vi "External Actuator Calibrations DAO.vi"(7 "refnum":T2, 8 "error in (no error)":errorcluster, 9 "External Actuator Id":T1, 10 "Actuator Calibrations":T3, 11 "Persistent DAO Actions":T4) -> (0 "error out":errorcluster, 2 "Actuator Settings Out":T3, 4 "refnum out":T2)   [LabVIEW 2009]
uses:
  Metadata/Persistant DAO Actions.ctl
  External Actuator Calibrations.ctl
  <vilib>/Utility/config.llb/Config Data RefNum.ctl
  External Actuator Id.ctl
  <vilib>/Utility/config.llb/Read Key (Double).vi
  <vilib>/Utility/config.llb/Write Key (Double).vi
  <vilib>/Utility/config.llb/NI_LVConfig.lvlib
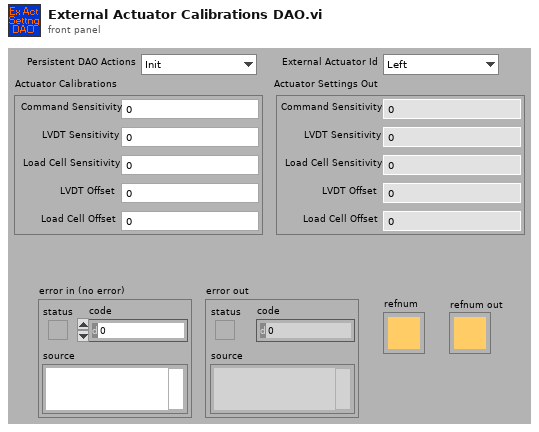
[diagram p1: front panel]
types:
  T1 = typedef "External Actuator Id.ctl" = enum16{"Left", "Right"}
  T2 = typedef "NI_LVConfig.lvlib/Config Data RefNum.ctl" = refnum<k1>
  T3 = typedef "External Actuator Calibrations.ctl" = cluster{"Load Cell Sensitivity":dbl, "Command Sensitivity":dbl, "LVDT Sensitivity":dbl, "LVDT Offset":dbl, "Load Cell Offset":dbl}
  T4 = typedef "Persistant DAO Actions.ctl" = enum16{"Init", "Get", "Set", "Load", "Save"}
  T5 = cluster{"Load Cell Sensitivity":dbl, "Command Sesntivity":dbl, "LVDT Sensitivity":dbl, "LVDT Offset":dbl, "Load Cell Offset":dbl}
  T6 = cluster{"Load Cell Sensitivity":dbl, "Command Sesntivity":dbl, "LVDT Sensitivity":dbl, "LVDT Offset":dbl, "Load Cell Offset":dbl}[]
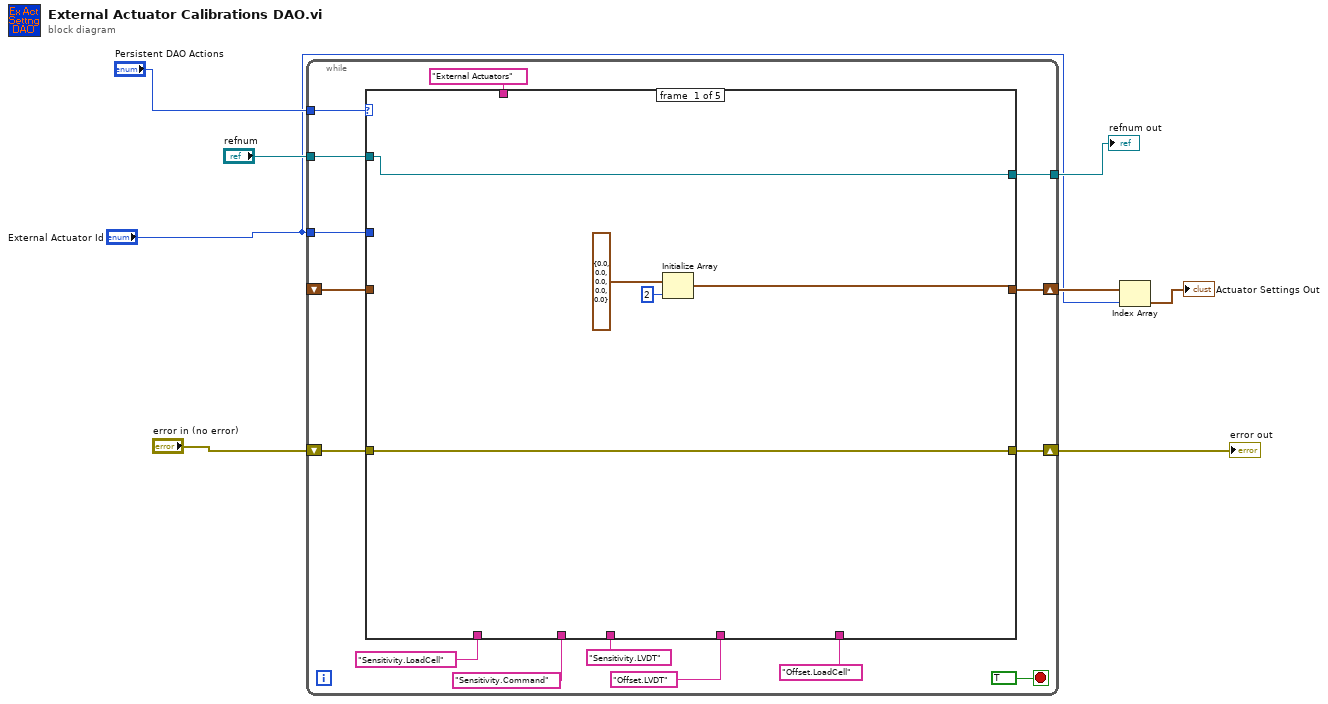
[diagram p0: block diagram]
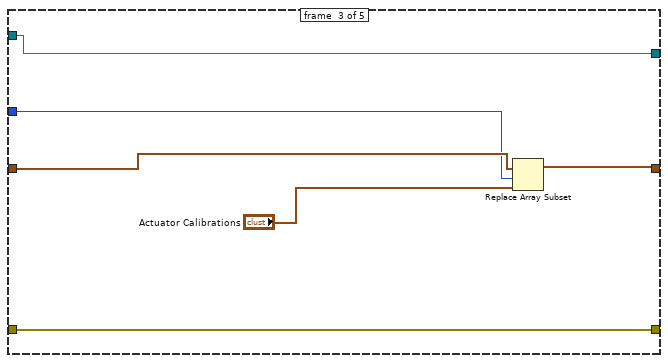
[diagram p3: hidden frame]
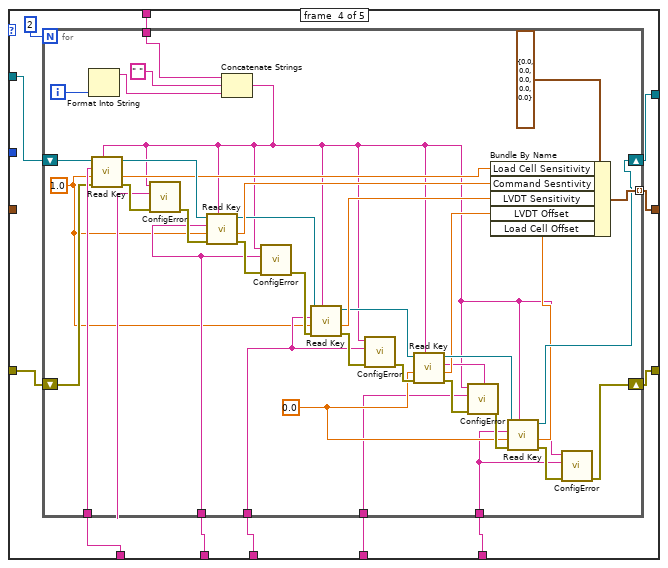
[diagram p4: hidden frame]
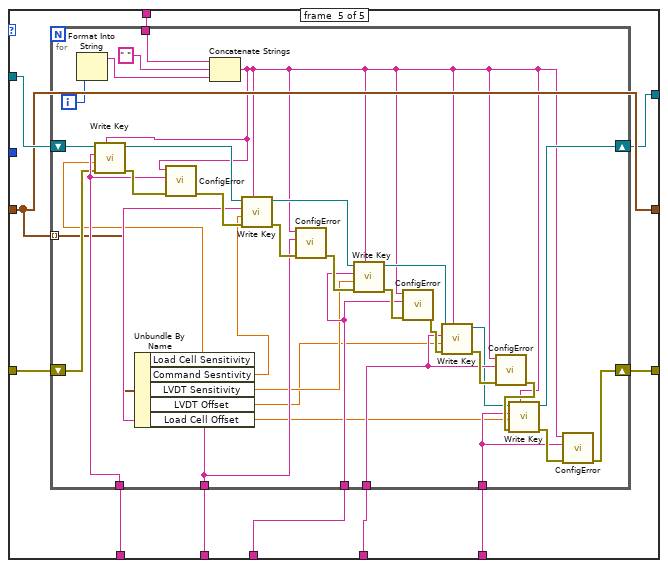
[diagram p5: hidden frame]
diagram:
  n1 = while {
    tunnel: "Persistent DAO Actions" -> [w22]
    shift-right: [w13] -> w7
    shift-left: _ -> [w14]
    tunnel: "refnum" -> [w19]
    shift-right: [w16] -> w4
    shift-left: "error in (no error)" -> [w17]
    tunnel: [w15] -> w3
    tunnel: "External Actuator Id" -> [w10]
    stop <- TRUE stop-if-true
    n2 = case shown="\"Save\"" w22 {
      tunnel: "External Actuators" -> [_ _ _ w41 w87]
      tunnel: "Sensitivity.LoadCell" -> [_ _ _ w49 w96]
      tunnel: w19 -> [w28 w30 w36 w48 w95]
      tunnel: "Sensitivity.Command" -> [_ _ _ w47 w94]
      tunnel: w17 -> [w27 w31 w37 w46 w93]
      tunnel: [w27 w31 w37 w42 w90] -> w16
      tunnel: [w28 w30 w36 w43 w88] -> w15
      tunnel: w14 -> [_ w29 w33 _ w92]
      tunnel: [w25 w29 w35 w40 w92] -> w13
      tunnel: "Sensitivity.LVDT" -> [_ _ _ w45 w91]
      tunnel: "Offset.LVDT" -> [_ _ _ w44 w89]
      tunnel: w10 -> [_ _ w32 _ _]
      tunnel: "Offset.LoadCell" -> [_ _ _ w38 w86]
      frame #0 {
        n3 = Initialize Array(T5 {"Load Cell Sensitivity"=0.0, "Command Sesntivity"=0.0, "LVDT Sensitivity"=0.0, "LVDT Offset"=0.0, "Load Cell Offset"=0.0} ("Autobalance Control In"), 2 ("dimension size")) -> (w25:T6)
      }
      frame #1 {
      }
      frame #2 {
        n4 = Replace Array Subset(array=w33, new element="Actuator Calibrations", index=w32) -> (w35:T6)
      }
      frame #3 {
        n5 = for {
          N: 2 -> [_]
          tunnel: w49 -> [w84]
          tunnel: w47 -> [w79]
          tunnel: w45 -> [w71]
          tunnel: w44 -> [w56]
          tunnel: w41 -> [w52]
          tunnel: [w66] -> w40 mode=indexing
          shift-right: [w60] -> w43
          shift-left: w48 -> [w83]
          shift-right: [w59] -> w42
          shift-left: w46 -> [w78]
          tunnel: w38 -> [w55]
          i -> [w50]
          w62 = 0.0
          w65 = 1.0 ("Port Number In")
          n6 = Format Into String(w50) -> (resulting string=w53:string)  [unwired: 3 in, 1 out]
          n7 = Concatenate Strings(w52, " " ("string"), w53) -> (w51:string)
          n8 = call-poly <vilib>:"Read Key.vi"("section"=w51, "error in (no error)"=w78, "default value"=w65, "key"=w84, "refnum"=w83) -> ("error out"=w85:errorcluster, "value"=w76:dbl, "refnum out"=w80:T2)  [unwired: 4 out]
          n9 = call "ConfigError.vi"("error in (no error)"=w85, "Key"=w84, "Section"=w51) -> ("error out"=w81:errorcluster)  [unwired: 8 out]
          n10 = call-poly <vilib>:"Read Key.vi"("section"=w51, "error in (no error)"=w81, "default value"=w65, "key"=w79, "refnum"=w80) -> ("error out"=w82:errorcluster, "value"=w75:dbl, "refnum out"=w73:T2)  [unwired: 4 out]
          n11 = call "ConfigError.vi"("error in (no error)"=w82, "Key"=w79, "Section"=w51) -> ("error out"=w72:errorcluster)  [unwired: 8 out]
          n12 = call-poly <vilib>:"Read Key.vi"("section"=w51, "error in (no error)"=w72, "default value"=w65, "key"=w71, "refnum"=w73) -> ("error out"=w74:errorcluster, "value"=w70:dbl, "refnum out"=w68:T2)  [unwired: 4 out]
          n13 = call "ConfigError.vi"("error in (no error)"=w74, "Key"=w71, "Section"=w51) -> ("error out"=w67:errorcluster)  [unwired: 8 out]
          n14 = call-poly <vilib>:"Read Key.vi"("section"=w51, "error in (no error)"=w67, "default value"=w62, "key"=w56, "refnum"=w68) -> ("error out"=w69:errorcluster, "value"=w58:dbl, "refnum out"=w61:T2)  [unwired: 4 out]
          n15 = call "ConfigError.vi"("error in (no error)"=w69, "Key"=w56, "Section"=w51) -> ("error out"=w63:errorcluster)  [unwired: 8 out]
          n16 = call-poly <vilib>:"Read Key.vi"("section"=w51, "error in (no error)"=w63, "default value"=w62, "key"=w55, "refnum"=w61) -> ("error out"=w64:errorcluster, "value"=w57:dbl, "refnum out"=w60:T2)  [unwired: 4 out]
          n17 = Bundle By Name(cluster=T5 {"Load Cell Sensitivity"=0.0, "Command Sesntivity"=0.0, "LVDT Sensitivity"=0.0, "LVDT Offset"=0.0, "Load Cell Offset"=0.0} ("Autobalance Control In"), "Load Cell Sensitivity"=w76, "Command Sesntivity"=w75, "LVDT Sensitivity"=w70, "LVDT Offset"=w58, "Load Cell Offset"=w57) -> (w66:T5)
          n18 = call "ConfigError.vi"("error in (no error)"=w64, "Key"=w55, "Section"=w51) -> ("error out"=w59:errorcluster)  [unwired: 8 out]
        }
      }
      frame #4 {
        n19 = for {
          tunnel: w96 -> [w128]
          tunnel: w94 -> [w123]
          tunnel: w92 -> [w121] mode=indexing
          tunnel: w91 -> [w115]
          tunnel: w89 -> [w111]
          tunnel: w87 -> [w101]
          shift-right: [w105] -> w88
          shift-left: w95 -> [w127]
          shift-right: [w106] -> w90
          shift-left: w93 -> [w122]
          tunnel: w86 -> [w103]
          i -> [w98]
          n20 = Format Into String(w98) -> (resulting string=w99:string)  [unwired: 3 in, 1 out]
          n21 = Unbundle By Name(w121) -> ("Load Cell Sensitivity"=w120:dbl, "Command Sesntivity"=w119:dbl, "LVDT Sensitivity"=w114:dbl, "LVDT Offset"=w110:dbl, "Load Cell Offset"=w102:dbl)
          n22 = Concatenate Strings(w101, " " ("string"), w99) -> (w100:string)
          n23 = call-poly <vilib>:"Write Key.vi"("section"=w100, "error in (no error)"=w122, "value"=w120, "key"=w128, "refnum"=w127) -> ("error out"=w129:errorcluster, "refnum out"=w124:T2)  [unwired: 3 in, 2 out]
          n24 = call "ConfigError.vi"("error in (no error)"=w129, "Key"=w128, "Section"=w100) -> ("error out"=w125:errorcluster)  [unwired: 8 out]
          n25 = call-poly <vilib>:"Write Key.vi"("section"=w100, "error in (no error)"=w125, "value"=w119, "key"=w123, "refnum"=w124) -> ("error out"=w126:errorcluster, "refnum out"=w116:T2)  [unwired: 3 in, 2 out]
          n26 = call "ConfigError.vi"("error in (no error)"=w126, "Key"=w123, "Section"=w100) -> ("error out"=w117:errorcluster)  [unwired: 8 out]
          n27 = call-poly <vilib>:"Write Key.vi"("section"=w100, "error in (no error)"=w117, "value"=w114, "key"=w115, "refnum"=w116) -> ("error out"=w118:errorcluster, "refnum out"=w109:T2)  [unwired: 3 in, 2 out]
          n28 = call "ConfigError.vi"("error in (no error)"=w118, "Key"=w115, "Section"=w100) -> ("error out"=w112:errorcluster)  [unwired: 8 out]
          n29 = call-poly <vilib>:"Write Key.vi"("section"=w100, "error in (no error)"=w112, "value"=w110, "key"=w111, "refnum"=w109) -> ("error out"=w113:errorcluster, "refnum out"=w104:T2)  [unwired: 3 in, 2 out]
          n30 = call "ConfigError.vi"("error in (no error)"=w113, "Key"=w111, "Section"=w100) -> ("error out"=w107:errorcluster)  [unwired: 8 out]
          n31 = call-poly <vilib>:"Write Key.vi"("section"=w100, "error in (no error)"=w107, "value"=w102, "key"=w103, "refnum"=w104) -> ("error out"=w108:errorcluster, "refnum out"=w105:T2)  [unwired: 3 in, 2 out]
          n32 = call "ConfigError.vi"("error in (no error)"=w108, "Key"=w103, "Section"=w100) -> ("error out"=w106:errorcluster)  [unwired: 8 out]
        }
      }
    }
  }
  "error out" <- w4
  "refnum out" <- w3
  n33 = Index Array(array=w7, index="External Actuator Id") -> (element=→"Actuator Settings Out":T5)
